vi "MPvPID_Determiner.vi"() -> ()   [LabVIEW 2020]
panel:
  out "Command State":T1(ring)
  in  "Target Arm State":T2(ring)
  in  "Previous Arm State":T2(ring)
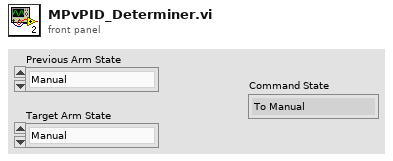
[diagram p1: front panel]
types:
  T1 = enum16{"To Manual", "From Manual", "Motion Profile", "PID Only"}
  T2 = enum16{"Manual", "High Cone", "High Cube", "Mid Cone", "Mid Cube", "Intake", "Cube Handoff", "Cone Handoff", "Stow"}
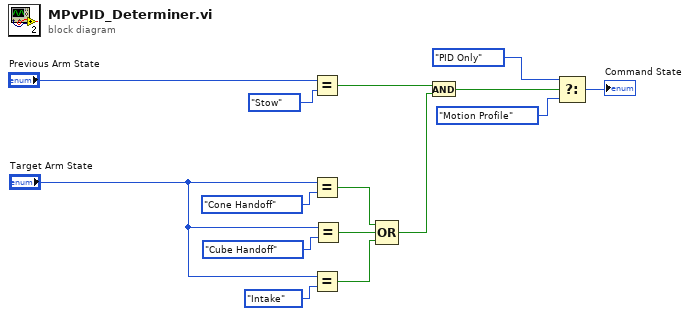
[diagram p0: block diagram]
diagram:
  n1 = Equal?(x="Previous Arm State", y=T2."Stow" ("Target Arm State 2")) -> (x = y?=w13:bool)
  n2 = Equal?(x="Target Arm State", y=T2."Cone Handoff" ("Target Arm State 2")) -> (x = y?=w9:bool)
  n3 = Equal?(x="Target Arm State", y=T2."Intake" ("Target Arm State 2")) -> (x = y?=w7:bool)
  n4 = Equal?(x="Target Arm State", y=T2."Cube Handoff" ("Target Arm State 2")) -> (x = y?=w8:bool)
  n5 = Compound Arithmetic op=OR(w9, w8, w7) -> (w6:bool)
  n6 = And(x=w13, y=w6) -> (x .and. y?=w5:bool)
  n7 = Select(t=T1."PID Only", s=w5, f=T1."Motion Profile") -> (s? t:f=→"Command State":T1)
